vi "Source V1 and V2.vi"(7 "Slew (V/s)":dbl=5.0, 8 "error in":errorcluster, 9 "V2 (V)":dbl, 10 "V1 (V)":dbl, 11 "VISA in":refnum<visa-resource-name>) -> (0 "error out":errorcluster, 3 "VISA out":refnum<visa-resource-name>)   [LabVIEW 2016, in "RP100.lvclass"]
uses:
  RP100.lvclass
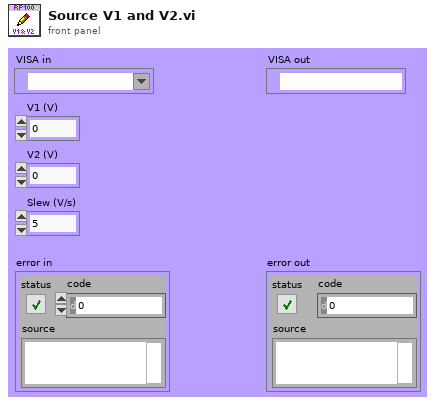
[diagram p1: front panel]
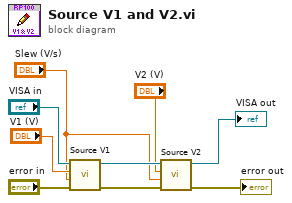
[diagram p0: block diagram]
diagram:
  n1 = call "Source V1.vi"("error in"="error in", "V1 rate"="Slew (V/s)", "V1"="V1 (V)", "VISA in"="VISA in") -> ("error out"=w8:errorcluster, "VISA out"=w9:refnum<visa-resource-name>)  [unwired: 4 in, 2 out]
  n2 = call "Source V2.vi"("error in"=w8, "V2 rate"="Slew (V/s)", "V2"="V2 (V)", "VISA in"=w9) -> ("error out"=→"error out":errorcluster, "VISA out"=→"VISA out":refnum<visa-resource-name>)  [unwired: 4 in, 2 out]
